vi "Edit_Server_Channel.vi"(5 "Mode":T1(ring)) -> ()   [LabVIEW 2010]
uses:
  Sub VIs/ADAM Controls/Ch_description_ADAM.ctl
  Sub VIs/ADAM Controls/Module_type_ADAM.ctl
  Sub VIs/ADAM Controls/Function_ADAM.ctl
  Sub VIs/ADAM Controls/Channel_State.ctl
  Sub VIs/ADAM Controls/Calib_type_ADAM.ctl
  Sub VIs/ADAM Controls/Address.ctl
  Sub VIs/ADAM Controls/Channel_names.ctl
panel:
  out "Help info":string
  in  "Search String":string
  out "Messages":string
  in  "Channel Names":i32(listbox)
  out "String Value":string
  in  "Numerical Value":dbl format="%.11f"
  in  "Ch Description":T2={"Ch Name"="", "Type"=enum."Test", "Function"=enum."Analogue Input", "Ch State"=enum."On", "Calibration type"=enum."Raw", "A"=0.0, "B"=0.0, "C"=0.0, "D"=0.0, "Comments"="", "Address"={"Main"=0, "Ch."=0, "Sub"=0, "Port Name"=""}, "String"="", "Duty"=65535} {"Duty" format="%.0b"; "D" format="%#_5g"; "C" format="%#_5g"; "B" format="%#_5g"; "A" format="%#_5g"}
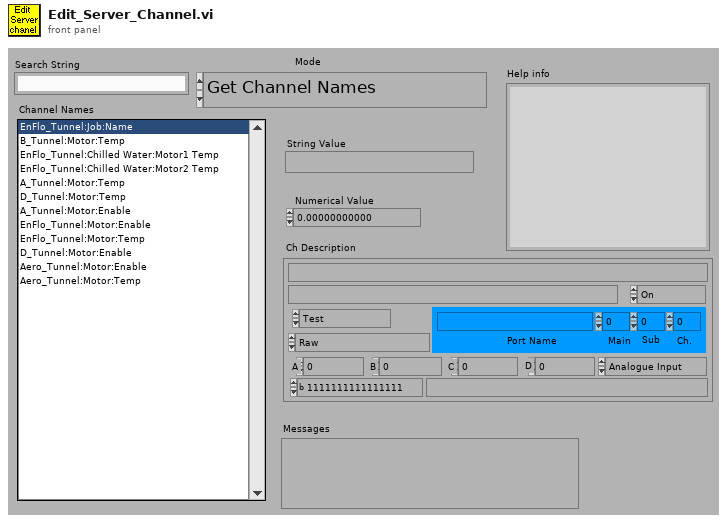
[diagram p1: front panel]
types:
  T1 = enum16{"Get Channel Names", "Get Current Value", "Update Channel Value", "Update Channel Description"}
  T2 = typedef "Ch_description_ADAM.ctl" = cluster{"Ch Name":string, "Type":T3, "Function":T4, "Ch State":T5, "Calibration type":T6, "A":dbl, "B":dbl, "C":dbl, "D":dbl, "Comments":string, "Address":T7, "String":string, "Duty":u16}
  T3 = typedef "Module_type_ADAM.ctl" = enum16{"4011", "4012", "4013", "4014", "4016", "4017", "4018", "4021", "4050", "4052", "4053", "4060", "4080", "5000", "5017", "5018", "5024", "5051", "5056", "5060", "6060", "Tracker", "WEST", "GILL", "JEM", "VICI", "Vaisala", "DRUCK", "Run VI Named:", "IR2100", "PPT", "Comparator", "VIRTUAL", "Hold Value", "Read A", "Read Ch", "Coded", "Client Info", "Web Client", "X10", "Test"}
  T4 = typedef "Function_ADAM.ctl" = enum16{"Analogue Input", "Digital Input", "Event counter", "Event rate", "Analogue Output", "Digital Output", "Relay Output"}
  T5 = typedef "Channel_State.ctl" = enum16{"On", "Off", "Always On", "Always Off"}
  T6 = typedef "Calib_type_ADAM.ctl" = enum16{"Raw", "Bx + A", "Cx^2 + Bx + A", "Dx^3 + Cx^2 + Bx + A", "In Band", "Hi-Tec Q", "Hi-Tec M_dot", "Text"}
  T7 = typedef "Address.ctl" = cluster{"Main":i32, "Ch.":i32, "Sub":i32, "Port Name":string}
  T8 = typedef "Channel_names.ctl" = enum16{"Active Only", "Active + Off", "All Channels"}
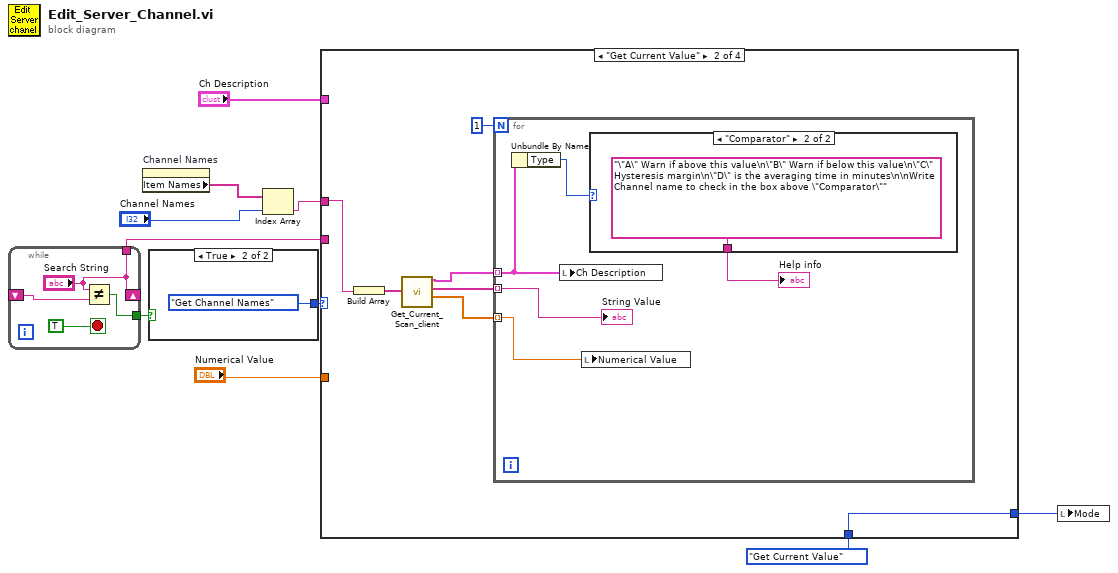
[diagram p0: block diagram]
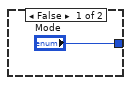
[diagram p2: hidden frame]
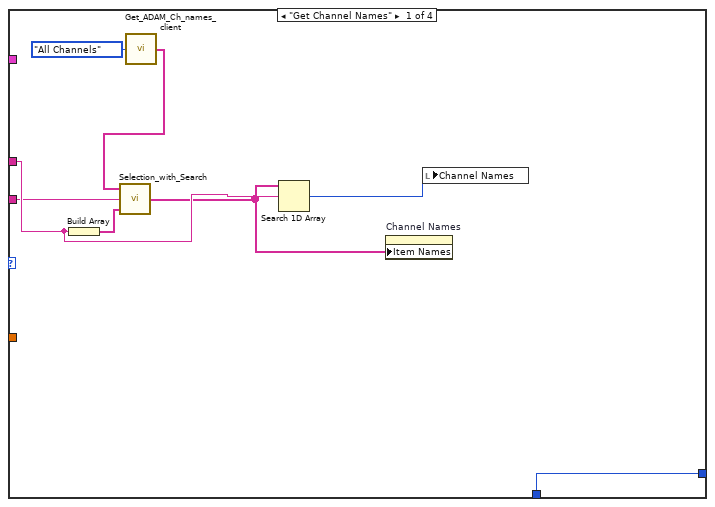
[diagram p3: hidden frame]
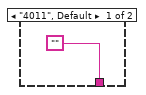
[diagram p4: hidden frame]
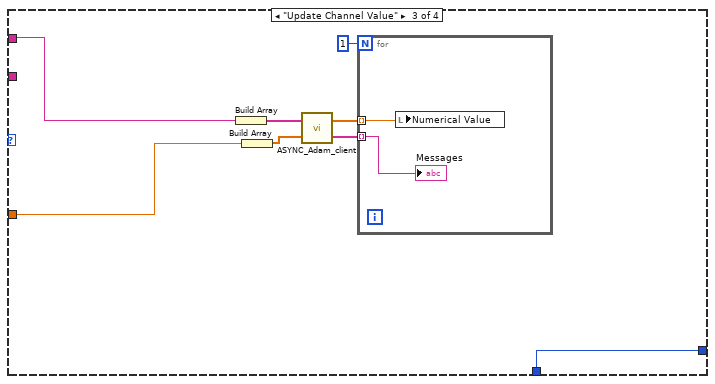
[diagram p5: hidden frame]
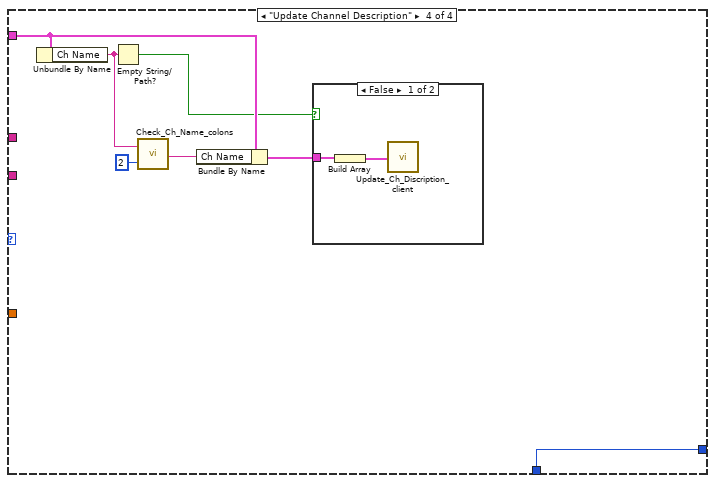
[diagram p6: hidden frame]
diagram:
  n1 = while {
    shift-right: ["Search String"] -> _
    shift-left: _ -> [w14]
    tunnel: [w13] -> w2
    tunnel: ["Search String"] -> w1
    stop <- TRUE stop-if-true
    n2 = Not Equal?(x="Search String", y=w14) -> (x != y?=w13:bool)
  }
  n3 = property on="Channel Names" class="LstBox (strict)"() -> ("Item Names"=w8:string[])  [unwired: 2 in, 2 out]
  n4 = case shown="True" w2 {
    tunnel: ["Mode" T1."Get Channel Names" ("Mode")] -> w10
    frame False {
    }
    frame True {
    }
  }
  n5 = Index Array(array=w8, index="Channel Names") -> (element=w7:string)
  n6 = case shown="\"Get Current Value\"" w10 {
    tunnel: w7 -> [w20 w30 w46 _]
    tunnel: "Numerical Value" -> [_ _ w43 _]
    tunnel: "Ch Description" -> [_ _ _ w54]
    tunnel: T1."Get Current Value" ("Mode") -> [w23 w25 w39 w55]
    tunnel: [w23 w25 w39 w55] -> w3
    tunnel: w1 -> [w17 _ _ _]
    frame "Get Channel Names" {
      n7 = Build Array(w20) -> (w21:string[])
      n8 = call "Get_ADAM_Ch_names_client.vi"("Channel names set"=Channel_names."All Channels") -> ("Ch names"=w22:string[])
      n9 = call "Selection_with_Search.vi"("Selected Channel Names"=w21, "Search String"=w17, "All Channel Names"=w22) -> ("Item Names"=w18:string[])
      n10 = Search 1D Array(1D array=w18, element=w20) -> (index of element=w19:i32)  [unwired: 1 out]
      n11 = property on="Channel Names" class="LstBox (strict)"("Item Names"=w18) -> ()  [unwired: 2 in, 2 out]
      n12 = local write "Channel Names"(w19) -> ()
    }
    frame "Get Current Value" {
      n13 = Build Array(w30) -> (w31:string[])
      n14 = call "Get_Current_Scan_client.vi"("ADAM Ch Names"=w31) -> ("Ch Description Array"=w28:T2[], "String values"=w27:string[], "Numerical Values"=w26:dbl[])  [unwired: 1 out]
      n15 = for {
        N: 1 -> [_]
        tunnel: w28 -> [w34] mode=indexing
        tunnel: w27 -> [w36] mode=indexing
        tunnel: w26 -> [w35] mode=indexing
        n16 = Unbundle By Name(w34) -> ("Type"=w33:T3)
        n17 = local write "Ch Description"(w34) -> ()
        n18 = local write "Numerical Value"(w35) -> ()
        n19 = case shown="\"Comparator\"" w33 {
          tunnel: ["" "\"A\" Warn if above this value\n\"B\" Warn if below this value\n\"C\" Hysteresis margin\n\"D\" is the averaging time in minutes\n\nWrite Channel name to check in the box above \"Comparator\""] -> w32
          frame "4011", Default {
          }
          frame "Comparator" {
          }
        }
        "Help info" <- w32
        "String Value" <- w36
      }
    }
    frame "Update Channel Value" {
      n20 = Build Array(w46) -> (w45:string[])
      n21 = Build Array(w43) -> (w44:dbl[])
      n22 = call "ASYNC_Adam_client.vi"("Values"=w44, "Channel Names"=w45) -> ("Scan Comments"=w40:string[], "Calibrated Units"=w41:dbl[])
      n23 = for {
        N: 1 -> [_]
        tunnel: w41 -> [w48] mode=indexing
        tunnel: w40 -> [w47] mode=indexing
        n24 = local write "Numerical Value"(w48) -> ()
        "Messages" <- w47
      }
    }
    frame "Update Channel Description" {
      n25 = Unbundle By Name(w54) -> ("Ch Name"=w53:string)
      n26 = Empty String/Path?(string/path=w53) -> (empty?=w49:bool)
      n27 = call "Check_Ch_Name_colons.vi"("No of Colons"=2, "Ch Name in"=w53) -> ("Ch Name out"=w51:string)
      n28 = Bundle By Name(cluster=w54, "Ch Name"=w51) -> (w50:T2)
      n29 = case shown="False" w49 {
        tunnel: w50 -> [w56 _]
        frame False {
          n30 = Build Array(w56) -> (w57:T2[])
          n31 = call "Update_Ch_Discription_client.vi"("Channels to update In"=w57) -> ()  [unwired: 1 out]
        }
        frame True {
        }
      }
    }
  }
  n32 = local write "Mode"(w3) -> ()
